vi "testcoil.vi"() -> ()   [LabVIEW 2020, in "PowerControl.lvlib"]
uses:
  Backup/PowerControl.lvlib
  Backup/YP03-60_Z/YP03-60_Z.lvclass
  Backup/YP03-60_X/YP03-60_X.lvclass
  Backup/YP03-60_Y/YP03-60_Y.lvclass
panel:
  in  "Zcoe":dbl[](array[numeric])=[3.4, 2.4, 1.4, 0.0, -1.4, -2.4, -3.4]
  in  "Ycoe":dbl[](array[numeric])=[3.4, 2.4, 1.4, 0.0, -1.4, -2.4, -3.4]
  in  "Xcoe":dbl[](array[numeric])=[5.0, 4.0, 3.0, 2.0, 1.0, 0.0, -1.0, -2.0, -3.0, -4.0, -5.0]
  in  "Array 3":dbl[](array[numeric])=[0.0, 1.4, 2.4, 3.4, 2.4, 1.4, 0.0, -1.4, -2.4, -3.4, -2.4, -1.4, 0.0, 1.4, 2.4, 3.4, 2.4, 1.4, 0.0]
  out "error out 4":errorcluster
  in  "error in (no error) 3":errorcluster
  in  "stop 3":bool
  out "error out 3":errorcluster
  in  "error in (no error) 2":errorcluster
  in  "stop 2":bool
  in  "Array 2":dbl[](array[numeric])=[0.0, 1.4, 2.4, 3.4, 2.4, 1.4, 0.0, -1.4, -2.4, -3.4, -2.4, -1.4, 0.0, 1.4, 2.4, 3.4, 2.4, 1.4, 0.0]
  in  "stop":bool
  out "error out 2":errorcluster
  in  "error in (no error)":errorcluster
  in  "Array":dbl[](array[numeric])=[0.0, 1.0, 2.0, 3.0, 4.0, 5.0, 4.0, 3.0, 2.0, 1.0, 0.0, -1.0, -2.0, -3.0, -4.0, -5.0, -4.0, -3.0, -2.0, -1.0, 0.0, 1.0, 2.0, 3.0, 4.0, 5.0, 4.0, 3.0, 2.0, 1.0, 0.0]
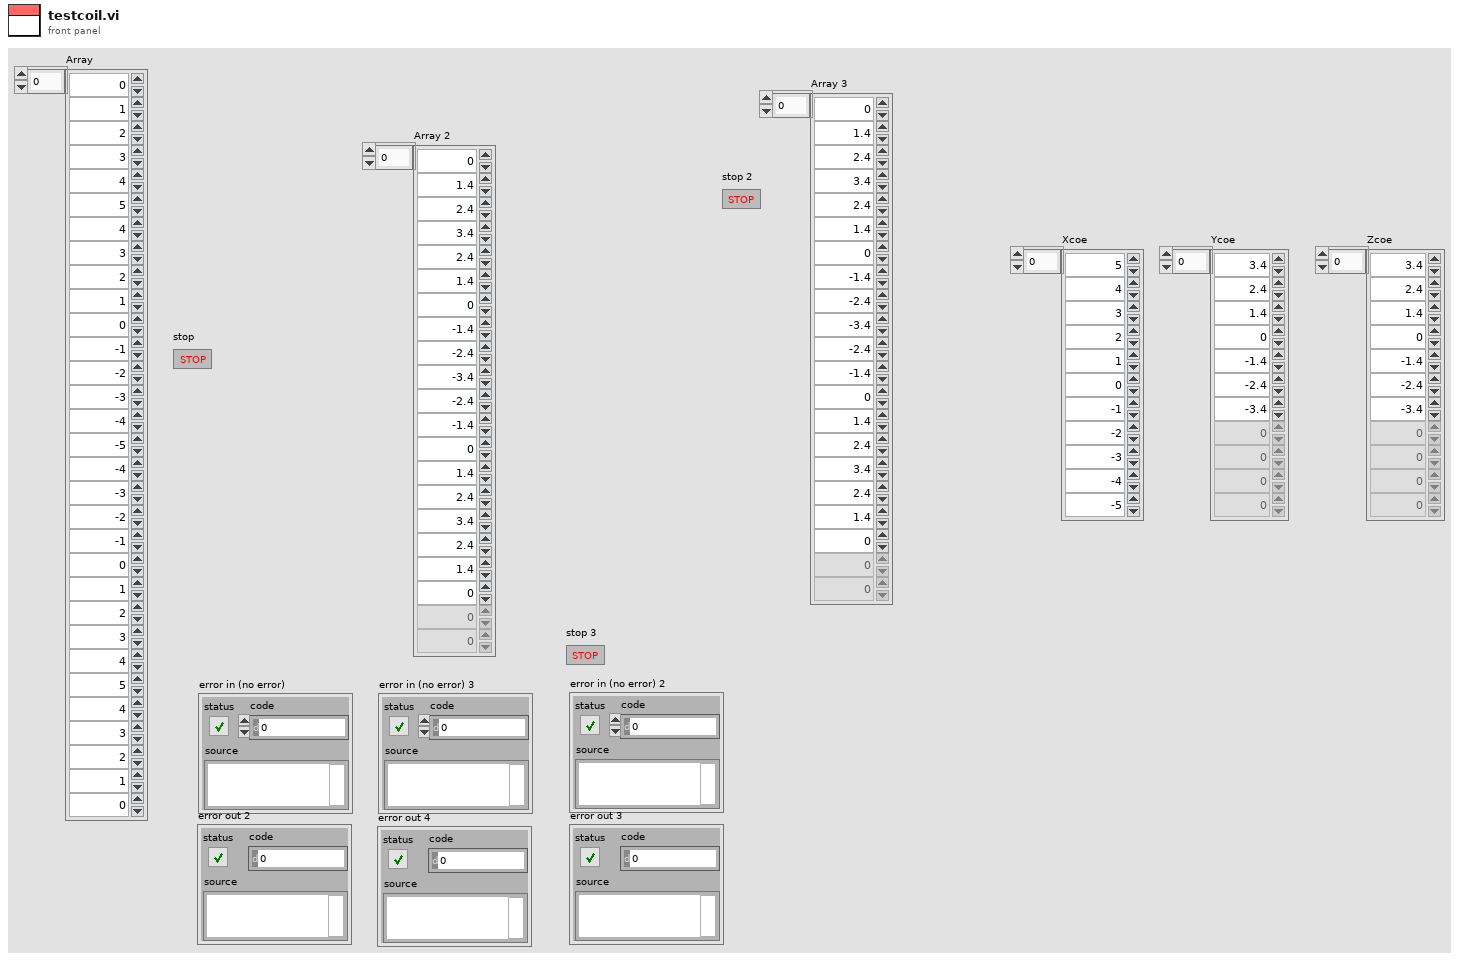
[diagram p1: front panel]
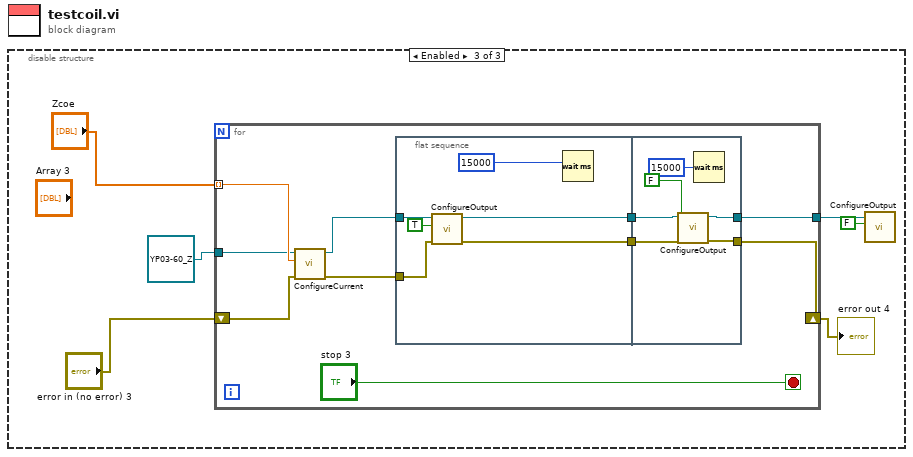
[diagram p0: block diagram]
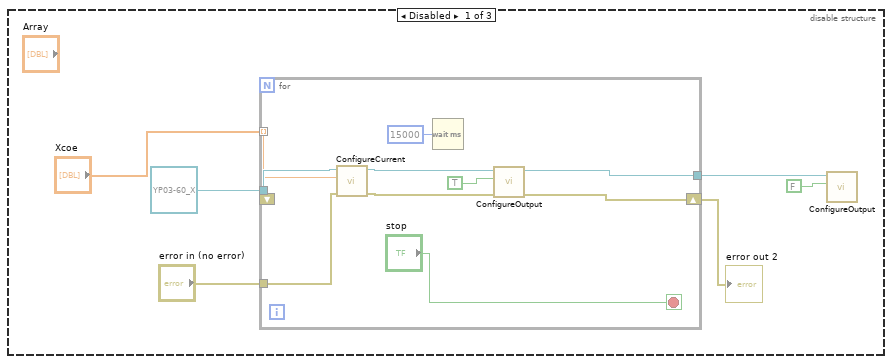
[diagram p2: hidden frame]
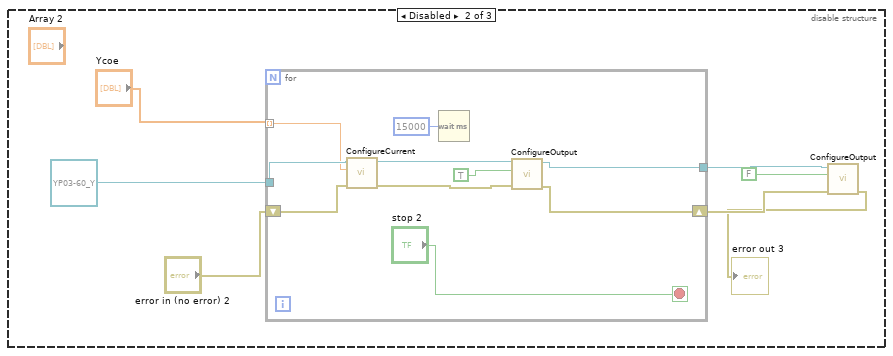
[diagram p3: hidden frame]
diagram:
  n1 = disable-structure shown="Enabled" {
    frame Disabled {
      n2 = for {
        tunnel: "Xcoe" -> [w9] mode=indexing
        tunnel: refnum<class "YP03-60_X.lvclass"> refnum ("PowerControl.lvlib:YP03-60_X.lvclass") -> [w16]
        tunnel: "error in (no error)" -> [w12]
        shift-right: [w14] -> w4
        shift-left: _ -> [_]
        tunnel: [w7] -> w3
        stop <- "stop" stop-if-true
        n3 = call-dynamic "ConfigureCurrent.vi"("error in (no error)"=w12, "Current(0)"=w9, "YP03-60_X in"=w16) -> ("error out 2"=w13:errorcluster, "YP03-60_X out"=w15:refnum<class "YP03-60_X.lvclass">)  [unwired: 7 in]
        n4 = Wait (ms)(milliseconds to wait=u32 15000) -> ()  [unwired: 1 out]
        n5 = call-dynamic "ConfigureOutput.vi"("error in (no error)"=w13, "Output((F)"=TRUE, "YP03-60_X in"=w15) -> ("error out 2"=w14:errorcluster, "YP03-60_X out"=w7:refnum<class "YP03-60_X.lvclass">)  [unwired: 7 in]
      }
      "error out 2" <- w4
      n6 = call-dynamic "ConfigureOutput.vi"("Output((F)"=FALSE, "YP03-60_X in"=w3) -> ()  [unwired: 8 in, 2 out]
    }
    frame Disabled {
      n7 = for {
        tunnel: "Ycoe" -> [w30] mode=indexing
        tunnel: refnum<class "YP03-60_Y.lvclass"> refnum ("PowerControl.lvlib:YP03-60_Y.lvclass") -> [w31]
        shift-right: [w25] -> w20
        shift-left: "error in (no error) 2" -> [w24]
        tunnel: [w26] -> w21
        stop <- "stop 2" stop-if-true
        n8 = call-dynamic "ConfigureCurrent.vi"("error in (no error)"=w24, "Current(0)"=w30, "YP03-60_Y in"=w31) -> ("error out"=w28:errorcluster, "YP03-60_Y out"=w29:refnum<class "YP03-60_Y.lvclass">)  [unwired: 7 in]
        n9 = Wait (ms)(milliseconds to wait=u32 15000) -> ()  [unwired: 1 out]
        n10 = call-dynamic "ConfigureOutput.vi"("error in (no error)"=w28, "Output((F)"=TRUE, "YP03-60_Y in"=w29) -> ("error out"=w25:errorcluster, "YP03-60_Y out"=w26:refnum<class "YP03-60_Y.lvclass">)  [unwired: 7 in]
      }
      n11 = call-dynamic "ConfigureOutput.vi"("error in (no error)"=w20, "Output((F)"=FALSE, "YP03-60_Y in"=w21) -> ("error out"=→"error out 3":errorcluster)  [unwired: 7 in, 1 out]
    }
    frame Enabled {
      n12 = for {
        tunnel: "Zcoe" -> [w49] mode=indexing
        tunnel: refnum<class "YP03-60_Z.lvclass"> refnum ("PowerControl.lvlib:YP03-60_Z.lvclass") -> [w48]
        shift-right: [w43] -> w37
        shift-left: "error in (no error) 3" -> [w45]
        tunnel: [w42] -> w36
        stop <- "stop 3" stop-if-true
        n13 = call-dynamic "ConfigureCurrent.vi"("error in (no error)"=w45, "Current(0)"=w49, "YP03-60_Z in"=w48) -> ("error out"=w46:errorcluster, "YP03-60_Z out"=w47:refnum<class "YP03-60_Z.lvclass">)  [unwired: 7 in]
        n14 = flat-sequence {
          tunnel: w47 -> [w55]
          tunnel: w46 -> [w53]
          tunnel: [w52] -> w41
          tunnel: [w51] -> w40
          tunnel: [w59] -> w42
          tunnel: [w57] -> w43
          tunnel: w41 -> [w58]
          tunnel: w40 -> [w60]
          frame #0 {
            n15 = call-dynamic "ConfigureOutput.vi"("error in (no error)"=w53, "Output((F)"=TRUE, "YP03-60_Z in"=w55) -> ("error out"=w52:errorcluster, "YP03-60_Z out"=w51:refnum<class "YP03-60_Z.lvclass">)  [unwired: 7 in]
            n16 = Wait (ms)(milliseconds to wait=u32 15000) -> ()  [unwired: 1 out]
          }
          frame #1 {
            n17 = call-dynamic "ConfigureOutput.vi"("error in (no error)"=w58, "Output((F)"=FALSE, "YP03-60_Z in"=w60) -> ("error out"=w57:errorcluster, "YP03-60_Z out"=w59:refnum<class "YP03-60_Z.lvclass">)  [unwired: 7 in]
            n18 = Wait (ms)(milliseconds to wait=u32 15000) -> ()  [unwired: 1 out]
          }
        }
      }
      "error out 4" <- w37
      n19 = call-dynamic "ConfigureOutput.vi"("Output((F)"=FALSE, "YP03-60_Z in"=w36) -> ()  [unwired: 8 in, 2 out]
    }
  }
